vi "Send SpectrumAcquired.vi"(7 "Message Priority (Normal)":T1=enum."Normal", 8 "error in (no error)":errorcluster, 10 "Spectrum":cluster{"Frequency":dbl[], "Amplitude":dbl[]}, 11 "Message Enqueuer":refnum<class "Message Enqueuer.lvclass">) -> (0 "error out":errorcluster, 3 "Message Enqueuer out":refnum<class "Message Enqueuer.lvclass">)   [LabVIEW 2023, in "SpectrumAnalyzerComm.lvlib" / "SpectrumAcquired Msg.lvclass"]
doc: "This VI sends the message to an actor."
uses:
  SpectrumAcquired Msg.lvclass
  <vilib>/ActorFramework/Message Enqueuer/Message Enqueuer.lvclass
  <vilib>/ActorFramework/Message Enqueuer/Message Priority.ctl
  C:/Program Files/National Instruments/LabVIEW 2023/vi.lib/ActorFramework/Message/Message.lvclass
  SpectrumAcquired Msg.lvclass/SpectrumAcquired Msg.ctl
  <vilib>/ActorFramework/Message Enqueuer/Message Enqueuer.lvclass/Message Enqueuer.ctl
  <vilib>/ActorFramework/Message Priority Queue/Priority Enqueue.vi
  C:/Users/Administrator/Documents/LVDAQ/Interfaces/AbstractInstrumentClasses/SpectrumAnalyzer_LV/SpectrumAnalyzerComm/SpectrumAnalyzerComm Messages/SpectrumAcquired Msg/SpectrumAcquired Msg.lvclass
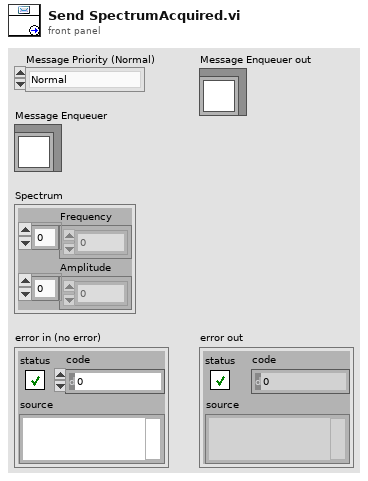
[diagram p1: front panel]
types:
  T1 = typedef "Actor Framework.lvlib/Message Enqueuer.lvclass/Message Priority.ctl" = enum16{"Low", "Normal", "High"}
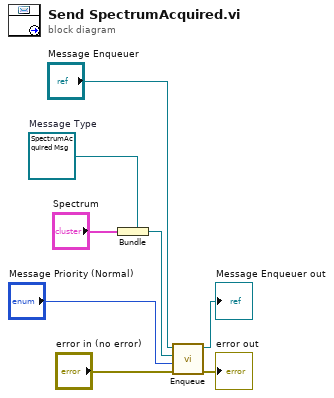
[diagram p0: block diagram]
diagram:
  w5 = refnum<class "SpectrumAcquired Msg.lvclass"> refnum  # Message Type
  n1 = Bundle(cluster=w5, "Spectrum") -> (w4:refnum<class "SpectrumAcquired Msg.lvclass">)
  n2 = call <vilib>:"Enqueue.vi"("error in (no error)"="error in (no error)", "Message Priority (Normal)"="Message Priority (Normal)", "Message"=w4, "Message Enqueuer in"="Message Enqueuer") -> ("error out"=→"error out":errorcluster, "Message Enqueuer in"=→"Message Enqueuer out":refnum<class "Message Enqueuer.lvclass">)  [unwired: 6 in]
